vi "LiquidFlow.vi"(8 "out_vol":dbl, 9 "in_vol":dbl, 10 "liquid":T2={"liquid_temperature"=array75x50[3750 elements], "water_level"=1.4948979591836733, "room_temperature"=298.15}, 11 "tank":T1) -> (1 "remainder_out_vol":dbl, 2 "remainder_in_vol":dbl, 3 "next_liquid":T2={"liquid_temperature"=array75x50[3750 elements], "water_level"=1.4948979591836733, "room_temperature"=298.15})   [LabVIEW 2020]
uses:
  Liquid.ctl
  TankResolution.ctl
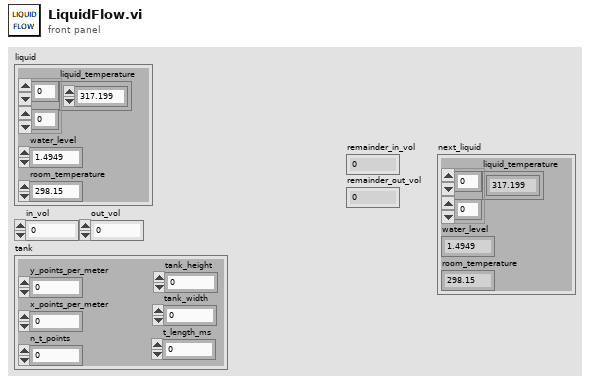
[diagram p1: front panel]
types:
  T1 = typedef "TankResolution.ctl" = cluster{"y_points_per_meter":i32, "x_points_per_meter":i32, "n_t_points":i32, "tank_height":dbl, "tank_width":dbl, "t_length_ms":u32}
  T2 = typedef "Liquid.ctl" = cluster{"liquid_temperature":dbl[][], "water_level":dbl, "room_temperature":dbl}
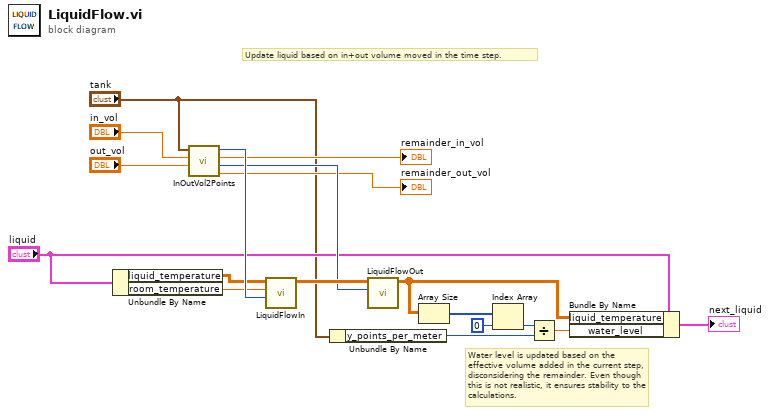
[diagram p0: block diagram]
diagram:
  # "Water level is updated based on the effective volume added in the current step, disconsidering the remainder. Even though this is not realistic, it ensures stability to the calculations."
  # "Update liquid based on in+out volume moved in the time step."
  n1 = Unbundle By Name("liquid") -> ("liquid_temperature"=w13:dbl[][], "room_temperature"=w12:dbl)
  n2 = call "InOutVol2Points.vi"("out_vol"="out_vol", "in_vol"="in_vol", "tank"="tank") -> ("remainder_out_vol"=→"remainder_out_vol":dbl, "out_points"=w16:i32, "remainder_in_vol"=→"remainder_in_vol":dbl, "in_points"=w17:i32)  [unwired: 5 in]
  n3 = call "LiquidFlowIn.vi"("level_increase_in_points"=w17, "room_temperature"=w12, "liquid_temperature"=w13) -> ("new_liquid_temperature"=w18:dbl[][])  [unwired: 8 in]
  n4 = Unbundle By Name("tank") -> ("y_points_per_meter"=w3:i32)
  n5 = call "LiquidFlowOut.vi"("level_decrease_in_points"=w16, "liquid_temperature"=w18) -> ("new_liquid_temperature"=w1:dbl[][])  [unwired: 9 in]
  n6 = Array Size(array=w1) -> (size(s)=w6:i32[])
  n7 = Index Array(array=w6, index=0) -> (element=w4:i32)
  n8 = Divide(x=w4, y=w3) -> (x/y=w2:dbl)
  n9 = Bundle By Name(cluster="liquid", "liquid_temperature"=w1, "water_level"=w2) -> (→"next_liquid":T2)
